vi "Add New Music.vi"(0 "reference in":refnum<class "MediaPlayer.lvclass">, 5 "Music Path":path, 11 "Error In":errorcluster) -> (4 "reference out":refnum<class "MediaPlayer.lvclass">, 15 "Error Out":errorcluster)   [LabVIEW 2024, in "MediaPlayer.lvclass"]
uses:
  MediaPlayer.lvclass
panel:
  # "Connector Pane"
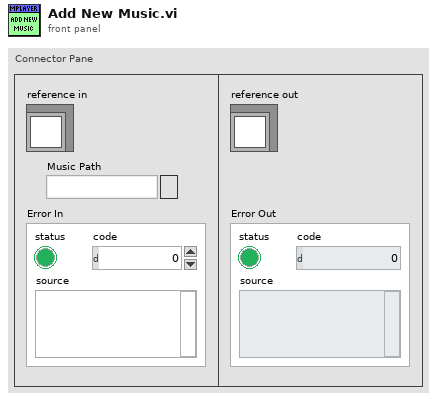
[diagram p1: front panel]
types:
  T1 = typedef "MediaPlayer.lvclass/ObjectAttributes.ctl" = cluster{"MediaPlayerData":T2, "Current Info":cluster{"Duration":dbl, "Name":string, "Is playing?":bool}}
  T2 = typedef "MediaPlayer.lvclass/MediaPlayer Data.ctl" = cluster{"Music List":path[], "Current Music Index":i64, "Song Handler":T3, "Device ID":u32}
  T3 = typedef "Sound Output Task ID.ctl" = u32
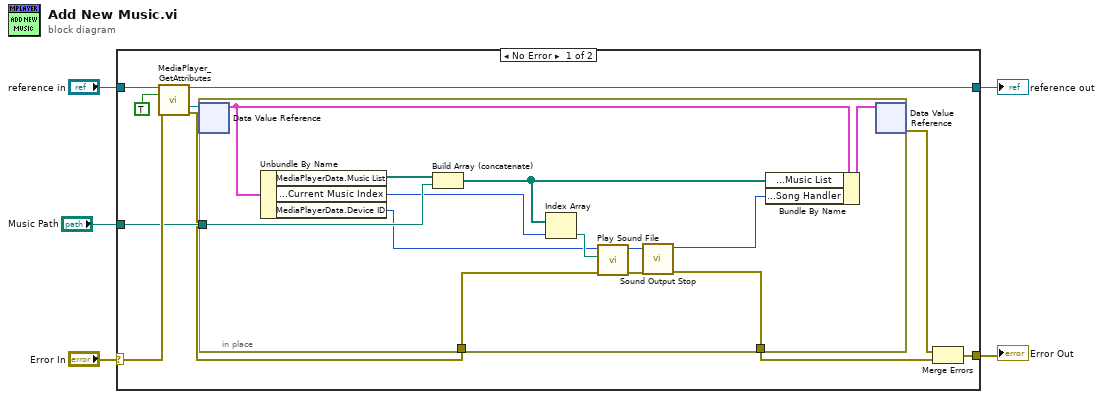
[diagram p0: block diagram]
diagram:
  n1 = case shown="No Error" "Error In" {
    selector: "Error In" -> [w14 w30]
    tunnel: [w7 w30] -> w4
    tunnel: [w13 w29] -> w2
    tunnel: "reference in" -> [w15 w29]
    tunnel: "Music Path" -> [w10 _]
    frame No Error {
      n2 = call "MediaPlayer_GetAttributes.vi"("reference in"=w15, "OnlyGetDvrReference(False)"=TRUE, "Error In"=w14) -> ("reference out"=w13:refnum<class "MediaPlayer.lvclass">, "DataRef"=w12:refnum<data-value>, "Error Out"=w8:errorcluster)  [unwired: 9 in, 1 out]
      n3 = in-place {
        in-place-border: w10 -> [w25]
        in-place-border: [w21] -> w9
        in-place-border: w8 -> [w18]
        n4 = in-place-dvr #1(w12) -> (w27:T1)  [unwired: 1 out]
        n5 = Unbundle By Name(w27) -> ("MediaPlayerData.Music List"=w26:path[], "MediaPlayerData.Current Music Index"=w17:i64, "MediaPlayerData.Device ID"=w16:u32)
        n6 = Build Array (concatenate)(w26, w25) -> (w20:path[])
        n7 = Index Array(array=w20, index=w17) -> (element=w23:path)
        n8 = call <vilib>:"Play Sound File.vi"("error in (no error)"=w18, "path"=w23, "device ID"=w16) -> ("error out"=w24:errorcluster, "task ID"=w19:T3)  [unwired: 7 in]
        n9 = call <vilib>:"Sound Output Stop.vi"("error in (no error)"=w24, "task ID"=w19) -> ("error out"=w21:errorcluster, "task ID out"=w22:T3)  [unwired: 8 in]
        n10 = Bundle By Name(cluster=w27, "MediaPlayerData.Music List"=w20, "MediaPlayerData.Song Handler"=w22) -> (w28:T1)
        n11 = in-place-dvr #1(w28) -> (w6:errorcluster)  [unwired: 1 out]
      }
      n12 = Merge Errors(w6, w9) -> (w7:errorcluster)
    }
    frame Error {
    }
  }
  "Error Out" <- w4
  "reference out" <- w2
